vi "Not Boolean Array (U32).vi"(4 "X":bool[](array[boolean])=[FALSE, FALSE, FALSE, FALSE, FALSE, FALSE, FALSE, TRUE, FALSE, FALSE, FALSE, FALSE, FALSE, FALSE, FALSE, FALSE, FALSE, FALSE, FALSE, FALSE, FALSE, FALSE, FALSE, FALSE, FALSE, FALSE, FALSE, FALSE, FALSE, FALSE, FALSE, FALSE]) -> (1 "Not X":bool[](array[boolean]))   [LabVIEW 2011]
doc: "This VI performs not operation on Boolean Array of Size 32"
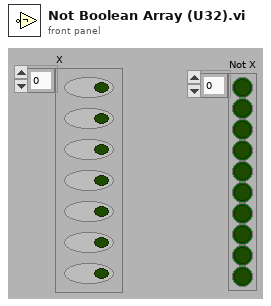
[diagram p1: front panel]
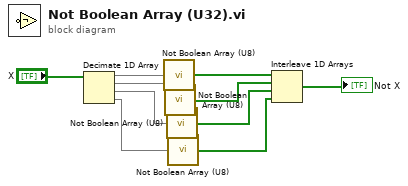
[diagram p0: block diagram]
diagram:
  n1 = Decimate 1D Array("X") -> (w9:bool[], w8:bool[], w7:bool[], w6:bool[])
  n2 = call <userlib>:"Not Boolean Array (U8).vi"("X"=w9) -> ("Not X"=w5:bool[])  [unwired: 4 in]
  n3 = call <userlib>:"Not Boolean Array (U8).vi"("X"=w8) -> ("Not X"=w4:bool[])  [unwired: 4 in]
  n4 = call <userlib>:"Not Boolean Array (U8).vi"("X"=w7) -> ("Not X"=w3:bool[])  [unwired: 4 in]
  n5 = call <userlib>:"Not Boolean Array (U8).vi"("X"=w6) -> ("Not X"=w2:bool[])  [unwired: 4 in]
  n6 = Interleave 1D Arrays(w5, w4, w3, w2) -> (→"Not X":bool[])
